vi "GUI.vi"(8 "error in":errorcluster, 11 "Electronic Load in":refnum<class "Electronic Load.lvclass">) -> (0 "error out":errorcluster, 3 "Electronic Load out":refnum<class "Electronic Load.lvclass">)   [LabVIEW 2019, in "Electronic Load.lvlib" / "Electronic Load.lvclass"]
uses:
  Electronic Load.lvclass
  Custom Controls/E-Load Mode.ctl
  Custom Controls/E-Load Function.ctl
  Custom Controls/Channel Select.ctl
panel:
  out "Handle":string
  out "E-Load Table":string[][](table)
  out "Delta(mS)":dbl
  in  "Continuous":bool
  in  "Set Trig":bool
  in  "Trigger":bool
  in  "Apply":bool
  in  "Function":T1
  in  "Select Channel":T3
  in  "stop":bool
  out "Waveform Graph":waveform(dbl)[](graph)
  out "Waveform Chart":waveform(dbl)[](graph)
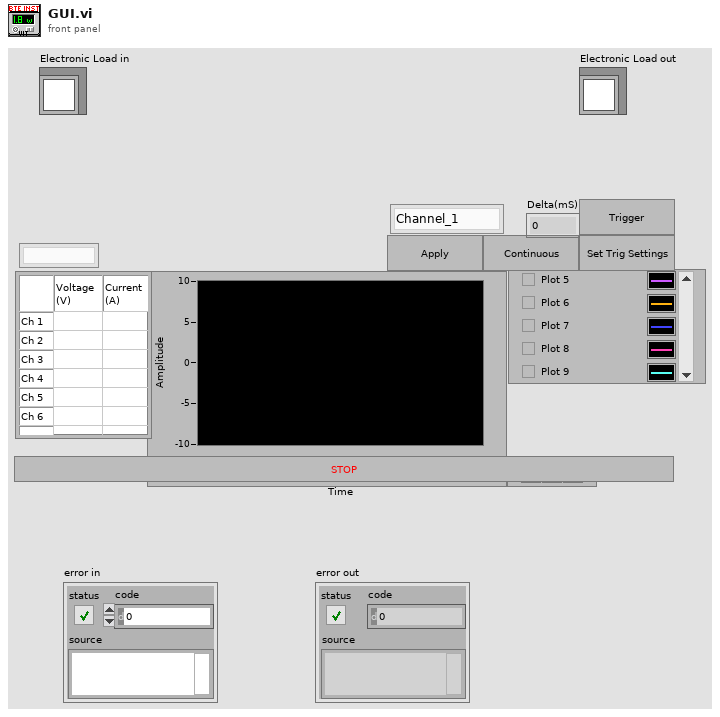
[diagram p1: front panel]
types:
  T1 = typedef "Electronic Load.lvlib/Electronic Load.lvclass/E-Load Function.ctl" = cluster{"Output":bool, "Slew Rate":dbl, "Mode":T2, "Input Level":dbl}
  T2 = typedef "Electronic Load.lvlib/Electronic Load.lvclass/E-Load Mode.ctl" = enum16{"Current", "Resistance", "Voltage"}
  T3 = typedef "Electronic Load.lvlib/Electronic Load.lvclass/Channel Select.ctl" = enum16{"Channel_1", "Channel_2", "Channel_3", "Channel_4", "Channel_5", "Channel_6"}
  T4 = cluster{"Total Current":waveform(dbl)[], "Current":waveform(dbl)[], "Voltage":waveform(dbl)[]}
  T5 = typedef "LVCursorListTypeDef.ctl" = cluster{"Name":string, "Color":u32, "Style":u8, "Point Style":u8, "Name Visible":bool, "Allow Drag":bool, "Cursor Mode":u32, "Plot":i32, "Index":i32, "Position":cluster{"X":dbl, "Y":dbl}, "X Scale":u32, "Y Scale":u32, "Watch Plots":i32[], "Watch All Plots":bool, "Plot Area":i32, "Label Offset":cluster{"X":dbl, "Y":dbl}}[]
  T6 = cluster{"Name":string, "Color":u32, "Style":u8, "Point Style":u8, "Name Visible":bool, "Allow Drag":bool, "Cursor Mode":u32, "Plot":i32, "Index":i32, "Position":cluster{"X":dbl, "Y":dbl}, "X Scale":u32, "Y Scale":u32, "Watch Plots":i32[], "Watch All Plots":bool, "Plot Area":i32, "Label Offset":cluster{"X":dbl, "Y":dbl}}
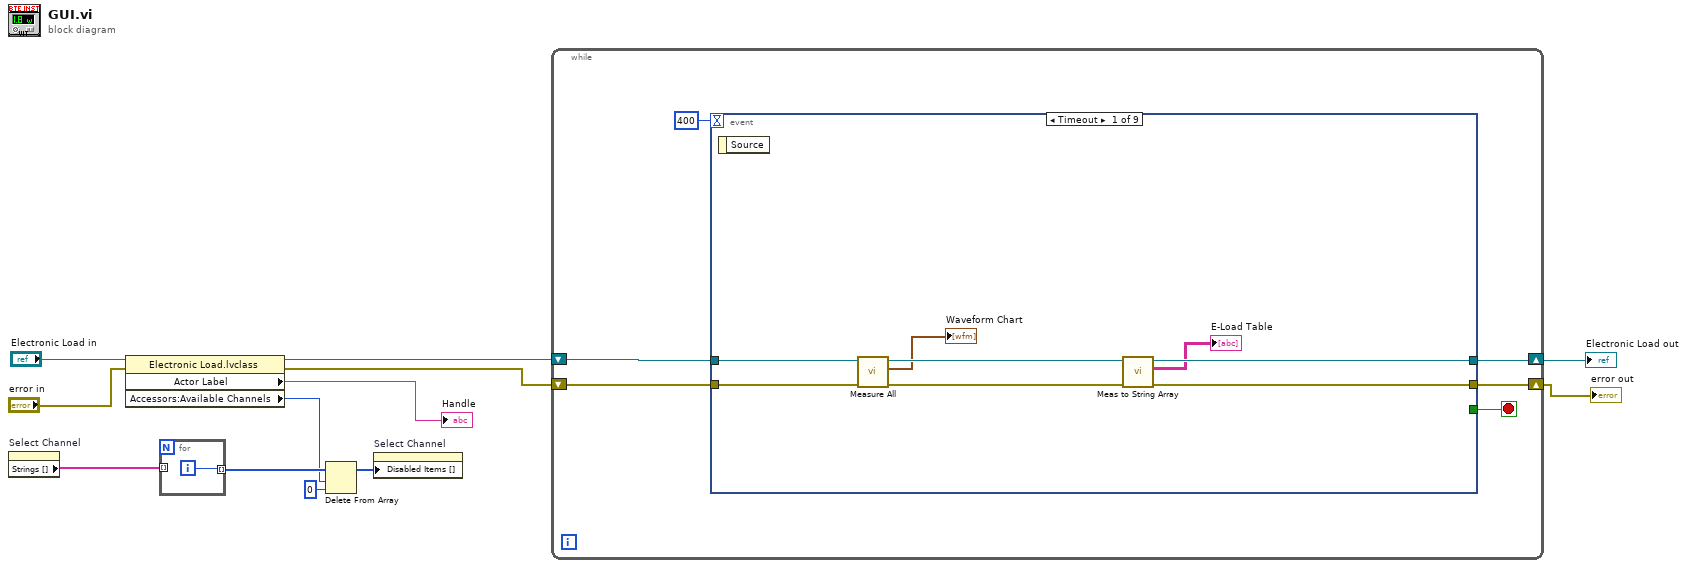
[diagram p0: block diagram]
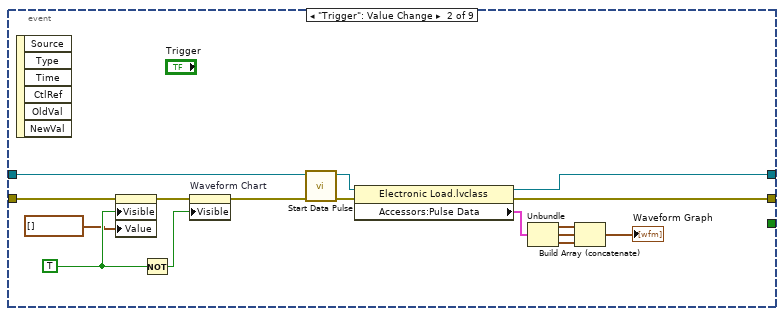
[diagram p2: hidden frame]
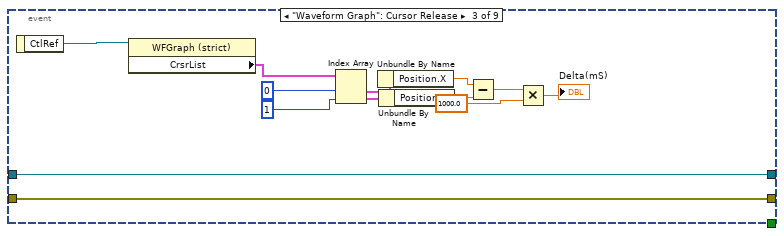
[diagram p3: hidden frame]
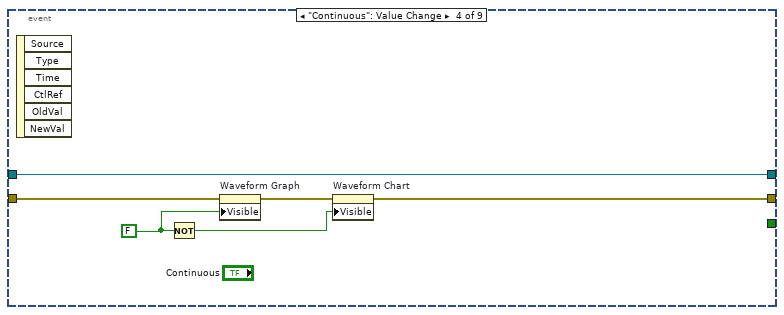
[diagram p4: hidden frame]
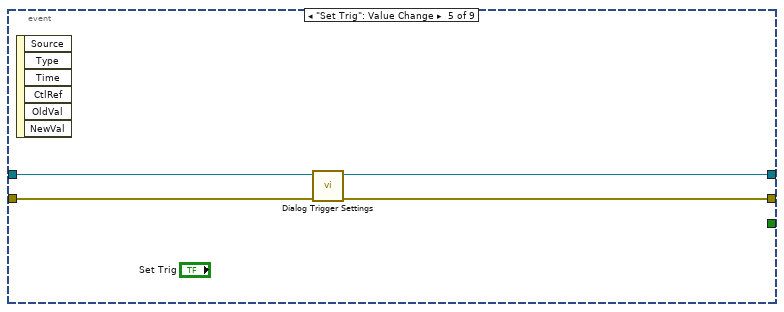
[diagram p5: hidden frame]
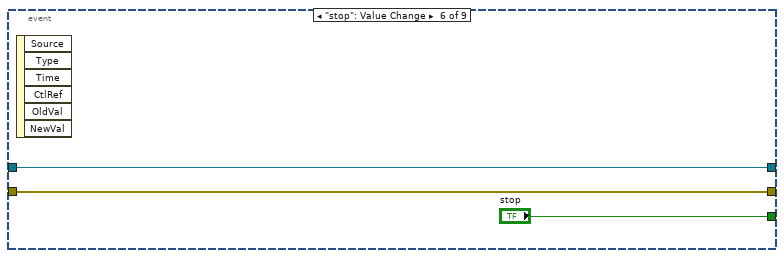
[diagram p6: hidden frame]
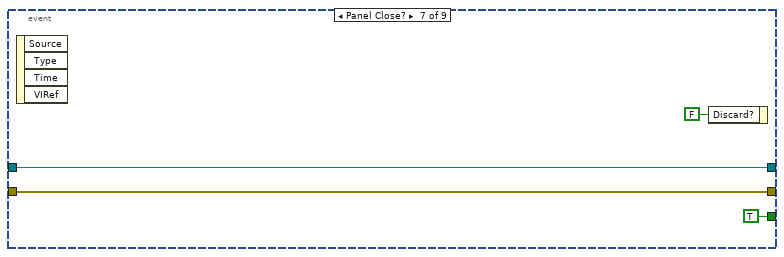
[diagram p7: hidden frame]
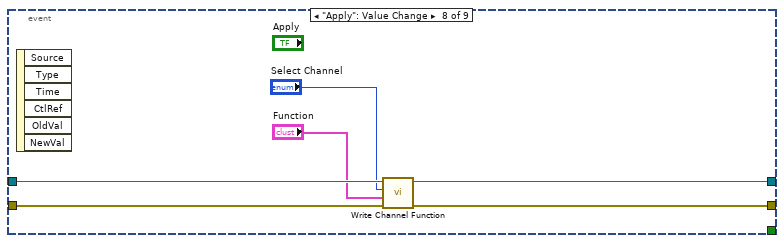
[diagram p8: hidden frame]
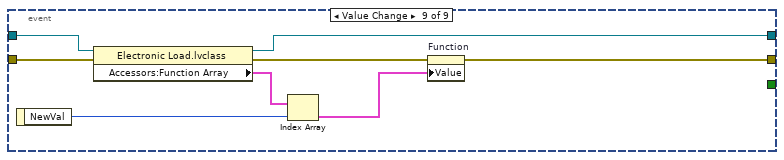
[diagram p9: hidden frame]
diagram:
  n1 = property on="Select Channel" class="Enum (strict)"() -> ("Strings []"=w12:string[])  [unwired: 2 in, 2 out]
  n2 = property class="Electronic Load.lvclass"(reference="Electronic Load in", error in="error in") -> (reference out=w6:refnum<class "Electronic Load.lvclass">, error out=w5:errorcluster, "Actor Label"=→"Handle":string, "Accessors:Available Channels"=w3:i32)
  n3 = for {
    tunnel: [w13] -> w10 mode=indexing
    tunnel: w12 -> [_] mode=indexing
    i -> [w13]
  }
  n4 = Delete From Array(array=w10, length=w3, index=0) -> (array with subset deleted=w11:i32[])  [unwired: 1 out]
  n5 = property on="Select Channel" class="Enum (strict)"("Disabled Items []"=w11) -> ()  [unwired: 2 in, 2 out]
  n6 = while {
    shift-right: [w15] -> w1
    shift-left: w5 -> [w19]
    shift-right: [w17] -> w8
    shift-left: w6 -> [w18]
    stop <- w16 stop-if-true
    n7 = event shown="[0] Timeout" {
      selector: _ -> [_ _ _ _ _ _ _ _ _]
      dyn-events: _ -> [_ _ _ _ _ _ _ _ _]
      timeout: 400 -> [_ _ _ _ _ _ _ _ _]
      tunnel: [w25 w34 w44 w57 w63 w68 w72 w76 w83] -> w15
      tunnel: w19 -> [w24 w43 w44 w62 w64 w68 w72 w77 w82]
      tunnel: w18 -> [w27 w40 w45 w61 w66 w69 w73 w79 w81]
      tunnel: [w26 w33 w45 w61 w65 w69 w73 w78 w80] -> w17
      tunnel: [_ _ _ _ _ "stop" TRUE ("stop") _ _] -> w16
      event Timeout {
        n8 = event-data() -> ()  [unwired: 1 in, 1 out]
        n9 = call-dynamic "Measure All.vi"("error in (no error)"=w24, "Electronic Load in"=w27) -> ("error out"=w23:errorcluster, "Measured"=→"Waveform Chart":waveform(dbl)[], "Electronic Load out"=w22:refnum<class "Electronic Load.lvclass">)  [unwired: 7 in]
        n10 = call "Meas to String Array.vi"("error in"=w23, "Electronic Load in"=w22) -> ("error out"=w25:errorcluster, "V-I Table"=→"E-Load Table":string[][], "Electronic Load out"=w26:refnum<class "Electronic Load.lvclass">)  [unwired: 7 in]
      }
      event "Trigger": Value Change {
        w42 = TRUE ("Visible")
        n11 = event-data() -> ()  [unwired: 1 in, 6 out]
        n12 = property on="Waveform Graph" class="WFGraph (strict)"(error in=w43, "Visible"=w42, "Value"=waveform(dbl)[] [] ("Waveform Graph")) -> (error out=w39:errorcluster)  [unwired: 1 in, 1 out]
        n13 = Not(x=w42) -> (.not. x?=w38:bool)
        n14 = property on="Waveform Chart" class="WFChart (strict)"(error in=w39, "Visible"=w38) -> (error out=w37:errorcluster)  [unwired: 1 in, 1 out]
        n15 = call-dynamic "Start Data Pulse.vi"("error in (no error)"=w37, "Electronic Load in"=w40) -> ("error out"=w35:errorcluster, "Electronic Load out"=w36:refnum<class "Electronic Load.lvclass">)  [unwired: 8 in]
        n16 = property class="Electronic Load.lvclass"(reference=w36, error in=w35) -> (reference out=w33:refnum<class "Electronic Load.lvclass">, error out=w34:errorcluster, "Accessors:Pulse Data"=w32:T4)
        n17 = Unbundle(w32) -> ("Total Current"=w31:waveform(dbl)[], "Current"=w30:waveform(dbl)[], "Voltage"=w29:waveform(dbl)[])
        n18 = Build Array (concatenate)(w31, w30, w29) -> (→"Waveform Graph":waveform(dbl)[])
      }
      event "Waveform Graph": Cursor Release {
        n19 = event-data() -> ("CtlRef"=w47:refnum<vi>)  [unwired: 1 in]
        n20 = property class="WFGraph (strict)"(reference=w47) -> ("CrsrList"=w46:T5)  [unwired: 1 in, 2 out]
        n21 = Index Array(array=w46, index #1=0 ("index"), index #2=1 ("index")) -> (element #1=w54:T6, element #2=w53:T6)
        n22 = Unbundle By Name(w54) -> ("Position.X"=w51:dbl)
        n23 = Unbundle By Name(w53) -> ("Position.X"=w52:dbl)
        n24 = Subtract(x=w51, y=w52) -> (x-y=w50:dbl)
        n25 = Multiply(x=w50, y=1000.0) -> (x*y=→"Delta(mS)":dbl)
      }
      event "Continuous": Value Change {
        w60 = FALSE ("Visible")
        n26 = event-data() -> ()  [unwired: 1 in, 6 out]
        n27 = Not(x=w60) -> (.not. x?=w59:bool)
        n28 = property on="Waveform Graph" class="WFGraph (strict)"(error in=w62, "Visible"=w60) -> (error out=w58:errorcluster)  [unwired: 1 in, 1 out]
        n29 = property on="Waveform Chart" class="WFChart (strict)"(error in=w58, "Visible"=w59) -> (error out=w57:errorcluster)  [unwired: 1 in, 1 out]
      }
      event "Set Trig": Value Change {
        n30 = event-data() -> ()  [unwired: 1 in, 6 out]
        n31 = call-dynamic "Dialog Trigger Settings.vi"("error in (no error)"=w64, "Electronic Load in"=w66) -> ("error out"=w63:errorcluster, "Electronic Load out"=w65:refnum<class "Electronic Load.lvclass">)  [unwired: 8 in]
      }
      event "stop": Value Change {
        n32 = event-data() -> ()  [unwired: 1 in, 6 out]
      }
      event Panel Close? {
        n33 = event-data() -> ()  [unwired: 1 in, 4 out]
        n34 = event-data("Discard?"=FALSE) -> ()  [unwired: 1 in, 1 out]
      }
      event "Apply": Value Change {
        n35 = event-data() -> ()  [unwired: 1 in, 6 out]
        n36 = call "Write Channel Function.vi"("error in"=w77, "Function"="Function", "Channel List"="Select Channel", "Electronic Load in"=w79) -> ("error out"=w76:errorcluster, "Electronic Load out"=w78:refnum<class "Electronic Load.lvclass">)  [unwired: 6 in]
      }
      event Value Change {
        n37 = event-data() -> ("NewVal"=w87:T3)  [unwired: 1 in]
        n38 = property class="Electronic Load.lvclass"(reference=w81, error in=w82) -> (reference out=w80:refnum<class "Electronic Load.lvclass">, error out=w84:errorcluster, "Accessors:Function Array"=w85:T1[])
        n39 = Index Array(array=w85, index=w87) -> (element=w86:T1)
        n40 = property on="Function" class="Clust (strict)"(error in=w84, "Value"=w86) -> (error out=w83:errorcluster)  [unwired: 1 in, 1 out]
      }
    }
  }
  "Electronic Load out" <- w8
  "error out" <- w1
